vi "DATA OUT (SubVI).vi"(0 "CODED DATA":dbl[][](array[numeric])) -> (1 "FULL GAME player 1":string[][](array[string]), 2 "FULL GAME player 2":string[][](array[string]))   [LabVIEW 2009]
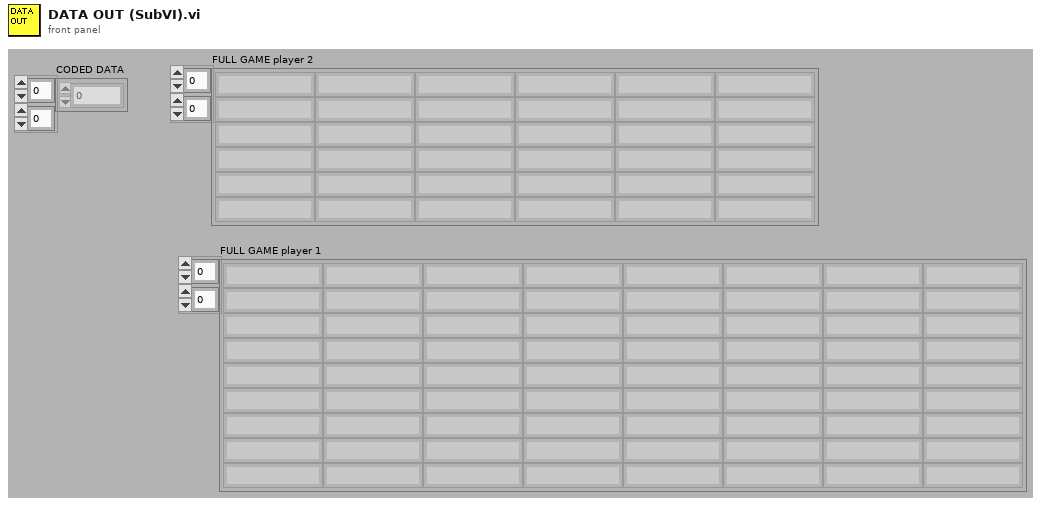
[diagram p1: front panel]
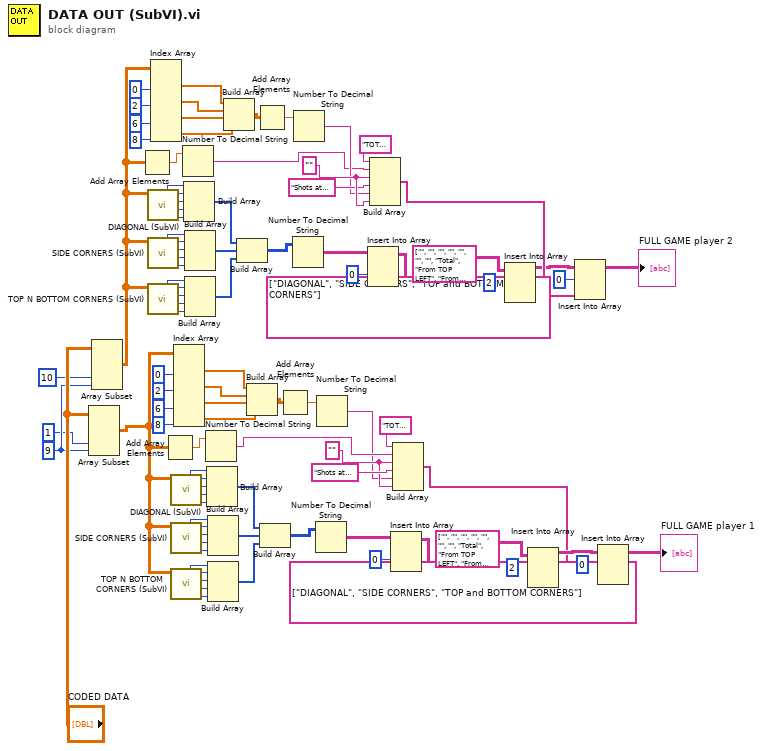
[diagram p0: block diagram]
diagram:
  w59 = ""
  w46 = ""
  w8 = 9 ("length")
  n1 = Array Subset(array="CODED DATA", index (col)=1 ("index"), length (col)=w8) -> (w5:dbl[][])  [unwired: 2 in]
  n2 = Array Subset(array="CODED DATA", index (col)=10 ("index"), length (col)=w8) -> (w96:dbl[][])  [unwired: 2 in]
  n3 = Add Array Elements(numeric array=w96) -> (sum=w39:dbl)
  n4 = call "DIAGONAL (SubVI).vi"("9 POSITION CODE"=w96) -> ("total"=w19:i32, "TL to BR"=w20:i32, "TR toBL"=w21:i32, "BL to TR"=w22:i32, "BR to TL"=w23:i32)  [unwired: 3 in]
  n5 = call "SIDE CORNERS (SubVI).vi"("9 POSITION CODE"=w96) -> ("total"=w24:i32, "TL to BL"=w25:i32, "TR toBR"=w26:i32, "BL to TL"=w27:i32, "BR to TR"=w28:i32)  [unwired: 3 in]
  n6 = call "TOP N BOTTOM CORNERS (SubVI).vi"("9 POSITION CODE"=w96) -> ("total"=w29:i32, "TL to TR"=w30:i32, "TR toTL"=w31:i32, "BL to BR"=w32:i32, "BR to BL"=w33:i32)  [unwired: 3 in]
  n7 = Index Array(array=w96, index (col) #1=0 ("disabled index (col)"), index (col) #2=2 ("index (col)"), index (col) #3=6 ("index (col)"), index (col) #4=8 ("index (col)")) -> (element #1=w18:dbl[], element #2=w15:dbl[], element #3=w16:dbl[], element #4=w17:dbl[])  [unwired: 4 in]
  n8 = Add Array Elements(numeric array=w5) -> (sum=w66:dbl)
  n9 = call "DIAGONAL (SubVI).vi"("9 POSITION CODE"=w5) -> ("total"=w86:i32, "TL to BR"=w85:i32, "TR toBL"=w84:i32, "BL to TR"=w83:i32, "BR to TL"=w82:i32)  [unwired: 3 in]
  n10 = call "SIDE CORNERS (SubVI).vi"("9 POSITION CODE"=w5) -> ("total"=w81:i32, "TL to BL"=w80:i32, "TR toBR"=w79:i32, "BL to TL"=w78:i32, "BR to TR"=w77:i32)  [unwired: 3 in]
  n11 = call "TOP N BOTTOM CORNERS (SubVI).vi"("9 POSITION CODE"=w5) -> ("total"=w76:i32, "TL to TR"=w75:i32, "TR toTL"=w74:i32, "BL to BR"=w73:i32, "BR to BL"=w72:i32)  [unwired: 3 in]
  n12 = Index Array(array=w5, index (col) #1=0 ("disabled index (col)"), index (col) #2=2 ("index (col)"), index (col) #3=6 ("index (col)"), index (col) #4=8 ("index (col)")) -> (element #1=w87:dbl[], element #2=w90:dbl[], element #3=w89:dbl[], element #4=w88:dbl[])  [unwired: 4 in]
  n13 = Number To Decimal String(number=w39) -> (decimal integer string=w1:string)  [unwired: 1 in]
  n14 = Build Array(w19, w20, w21, w22, w23) -> (w34:i32[])
  n15 = Build Array(w24, w25, w26, w27, w28) -> (w35:i32[])
  n16 = Build Array(w29, w30, w31, w32, w33) -> (w36:i32[])
  n17 = Number To Decimal String(number=w66) -> (decimal integer string=w4:string)  [unwired: 1 in]
  n18 = Build Array(w86, w85, w84, w83, w82) -> (w71:i32[])
  n19 = Build Array(w81, w80, w79, w78, w77) -> (w70:i32[])
  n20 = Build Array(w76, w75, w74, w73, w72) -> (w69:i32[])
  n21 = Build Array(w18, w15, w16, w17) -> (w14:dbl[][])
  n22 = Build Array(w34, w35, w36) -> (w37:i32[][])
  n23 = Build Array(w87, w90, w89, w88) -> (w91:dbl[][])
  n24 = Add Array Elements(numeric array=w14) -> (sum=w38:dbl)
  n25 = Build Array(w71, w70, w69) -> (w68:i32[][])
  n26 = Add Array Elements(numeric array=w91) -> (sum=w67:dbl)
  n27 = Number To Decimal String(number=w37) -> (decimal integer string=w43:string[][])  [unwired: 1 in]
  n28 = Number To Decimal String(number=w38) -> (decimal integer string=w2:string)  [unwired: 1 in]
  n29 = Number To Decimal String(number=w68) -> (decimal integer string=w62:string[][])  [unwired: 1 in]
  n30 = Number To Decimal String(number=w67) -> (decimal integer string=w3:string)  [unwired: 1 in]
  n31 = Insert Into Array(array=w43, index (col)=0 ("disabled index (col)"), new element=string[][] [["DIAGONAL"], ["SIDE CORNERS"], ["TOP and BOTTOM CORNERS"]]) -> (w48:string[][])  [unwired: 1 in]
  n32 = Build Array("TOTAL Shots by player", w1, w46, "Shots at the corner position", w2, w46) -> (w51:string[])
  n33 = Insert Into Array(array=w62, index (col)=0 ("disabled index (col)"), new element=string[][] [["DIAGONAL"], ["SIDE CORNERS"], ["TOP and BOTTOM CORNERS"]]) -> (w57:string[][])  [unwired: 1 in]
  n34 = Build Array("TOTAL Shots by player", w4, w59, "Shots at the corner position", w3, w59) -> (w54:string[])
  n35 = Insert Into Array(array=string[][] [["", "", "", "", "", ""], ["", "Total", "From TOP LEFT", "From TOP RIGHT", "From BOTTOM LEFT", "From BOTTOM RIGHT"]], index (row)=2, new element=w48) -> (w50:string[][])  [unwired: 1 in]
  n36 = Insert Into Array(array=string[][] [["", "", "", "", "", ""], ["", "Total", "From TOP LEFT", "From TOP RIGHT", "From BOTTOM LEFT", "From BOTTOM RIGHT"]], index (row)=2, new element=w57) -> (w55:string[][])  [unwired: 1 in]
  n37 = Insert Into Array(array=w50, index (row)=0, new element=w51) -> (→"FULL GAME player 2":string[][])  [unwired: 1 in]
  n38 = Insert Into Array(array=w55, index (row)=0, new element=w54) -> (→"FULL GAME player 1":string[][])  [unwired: 1 in]
